vi "DriveSystem.vi"() -> ()   [LabVIEW 2025]
panel:
  out "SwerveDrive/omegaActual":dbl caption="Vel Rot" format="%11.2f"
  out "SwerveDrive/vyActual":dbl caption="Vel Y" format="%12.1f"
  out "SwerveDrive/vyTarget":dbl caption="Vel Y Dmd" format="%12.1f"
  out "SwerveDrive/vxActual":dbl caption="Vel X" format="%12.1f"
  out "SwerveDrive/vxTarget":dbl caption="Vel X Dmd" format="%12.1f"
  out "SwerveDrive/GyroYaw":dbl caption="Gyro Yaw" format="%12.1f"
  out "SwerveDrive/GyroRoll":dbl caption="Gyro Roll" format="%12.1f"
  out "SwerveDrive/omegaTarget":dbl caption="Vel Rot Dmd" format="%11.2f"
  out "SwerveDrive/GyroPitch":dbl caption="Gyro Pitch" format="%12.1f"
  out "SwerveDrive/GyroConnected":bool caption="Gyro Connected"
  # "DRIVE"
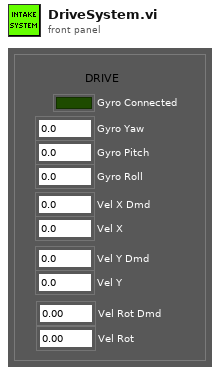
[diagram p1: front panel]
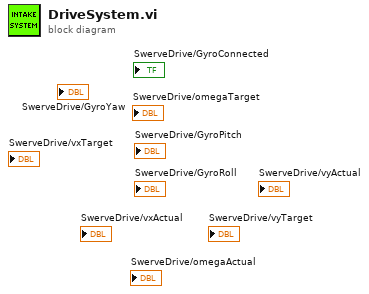
[diagram p0: block diagram]
diagram:
